vi "test.vi"() -> ()   [LabVIEW 2010]
uses:
  XImage/XImage.xctl
  classes/ImageCollection/ImageCollection/ImageCollection.lvclass
  XImage/ROI_mode_enum.ctl
  XImage/overlays_cluster.ctl
panel:
  in  "point radius":i32=5
  in  "Overlay":T1={"overlay array"=[{[[10, 10], [20, 30], [12, 45]]}], "overlay name"="test", "color (red)"=16711680, "overlay size"=3, "overlay type"=enum."crosshair"} {"overlay size" min=1}
  in  "size":cluster{"Width":u32, "Height":u32}
  in  "ROI mode":T2=enum."IMAQROIs"
  in  "overlay name":string
  in  "button:clear overlay":bool
  out "successful save?":bool
  in  "button:save ROIs":bool
  in  "button:load ROIs":bool
  in  "button:load image":bool
  out "has image loaded?":bool
  in  "enable numbering?":bool
  in  "ROI colour":u32(colorbox)=6618880
  in  "ROI Tools Palette visible":T3={"Zoom Tool"=TRUE, "Selection Tool"=TRUE, "Pan Tool"=TRUE, "Point Tool"=TRUE, "Line Tool"=TRUE, "Rectangle Tool"=TRUE, "Rotated Rectangle Tool"=TRUE, "Polyline Tool"=TRUE, "Polygon Tool"=TRUE, "Freehand Tool"=TRUE, "Closed Freehand Tool"=TRUE, "Ellipse Tool"=TRUE, "Annulus Tool"=TRUE}
  out "number of ROIs":i32
  in  "current frame index":i32
  out "number of images":i32
  in  "stop":bool
  in  "XImage":refnum<class "ImageCollection.lvclass">(xcontrol)
  # "Test panel for XImage"
  # "Overlay"
  # "ROIs"
  # "PointCollection"
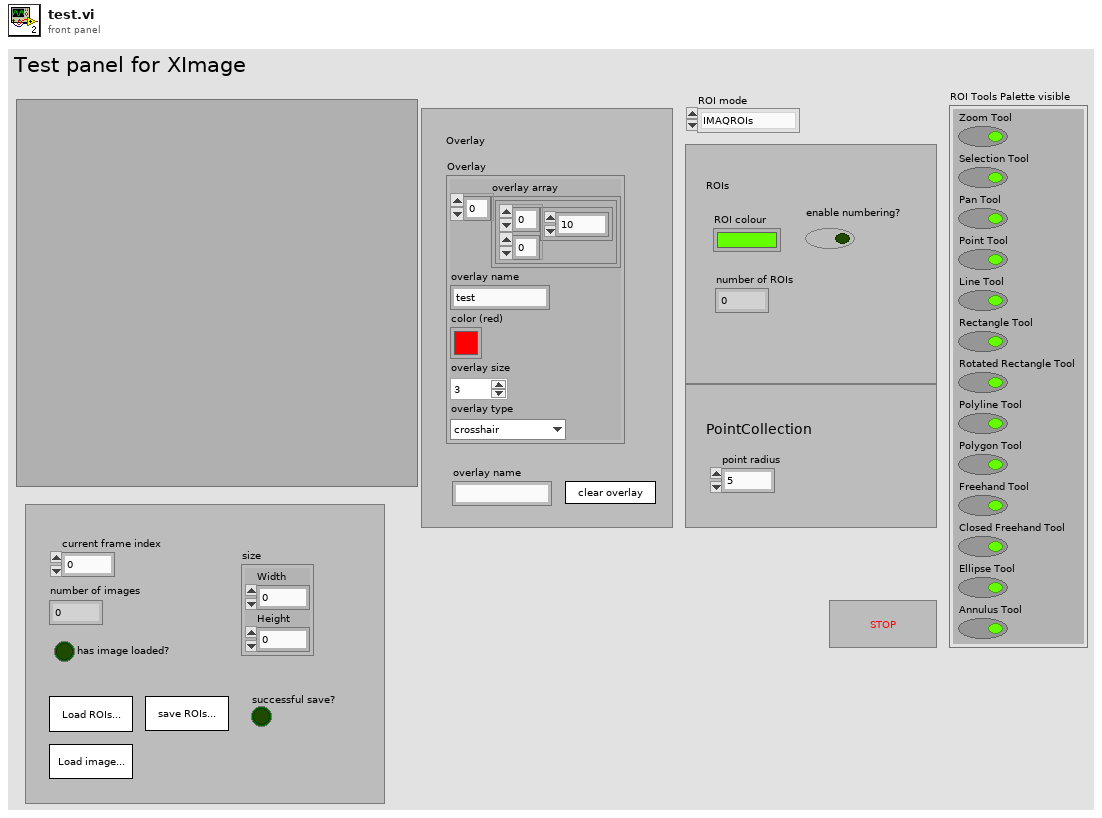
[diagram p1: front panel]
types:
  T1 = typedef "XImage.xctl/overlays_cluster.ctl" = cluster{"overlay array":cluster{i32[][]}[], "overlay name":string, "color (red)":u32, "overlay size":i32, "overlay type":enum16{"crosshair", "circle"}}
  T2 = typedef "XImage.xctl/ROI_mode_enum.ctl" = enum16{"none", "IMAQROIs", "PointCollection"}
  T3 = cluster{"Zoom Tool":bool, "Selection Tool":bool, "Pan Tool":bool, "Point Tool":bool, "Line Tool":bool, "Rectangle Tool":bool, "Rotated Rectangle Tool":bool, "Polyline Tool":bool, "Polygon Tool":bool, "Freehand Tool":bool, "Closed Freehand Tool":bool, "Ellipse Tool":bool, "Annulus Tool":bool}
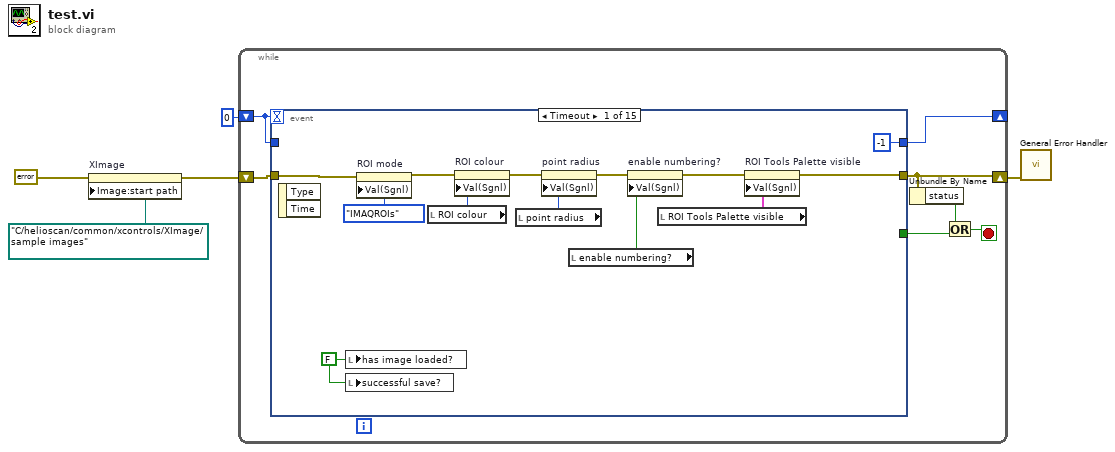
[diagram p0: block diagram]
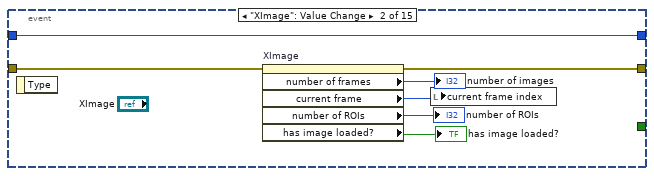
[diagram p2: hidden frame]
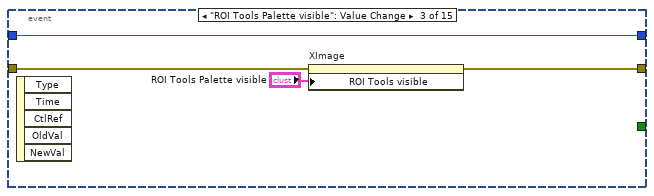
[diagram p3: hidden frame]
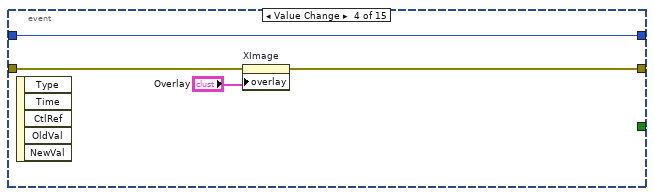
[diagram p4: hidden frame]
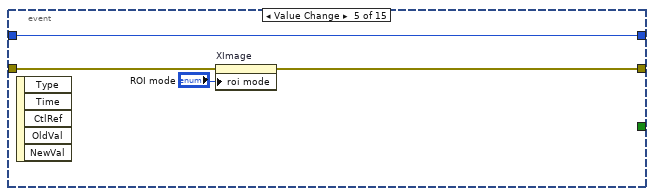
[diagram p5: hidden frame]
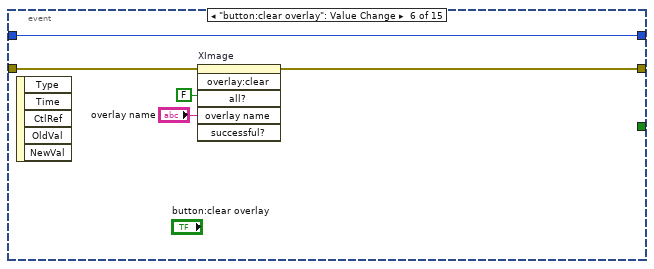
[diagram p6: hidden frame]
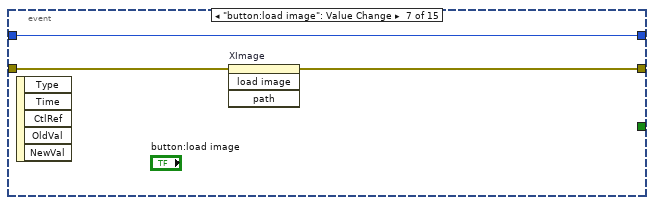
[diagram p7: hidden frame]
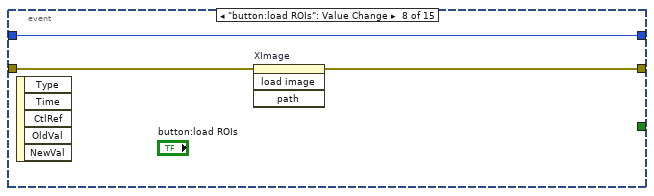
[diagram p8: hidden frame]
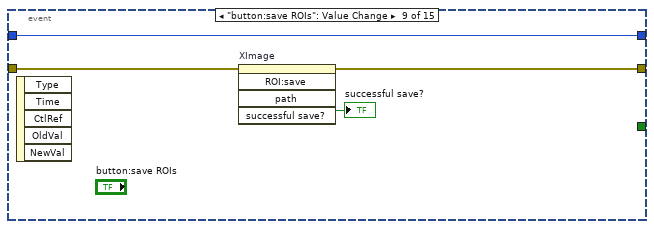
[diagram p9: hidden frame]
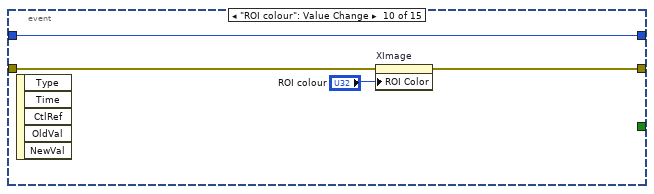
[diagram p10: hidden frame]
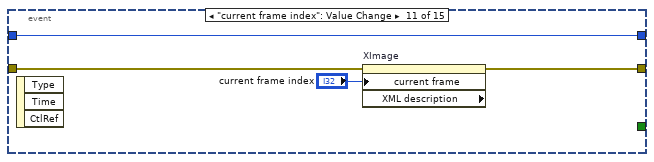
[diagram p11: hidden frame]
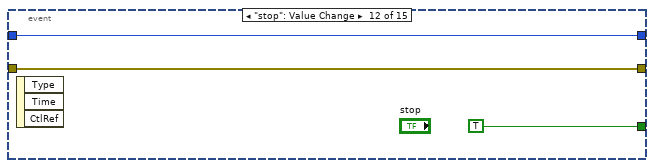
[diagram p12: hidden frame]
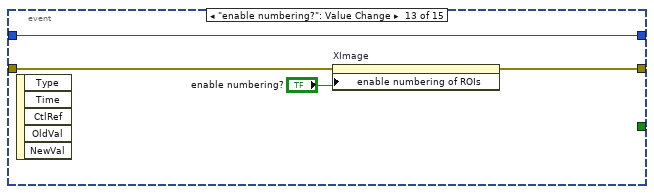
[diagram p13: hidden frame]
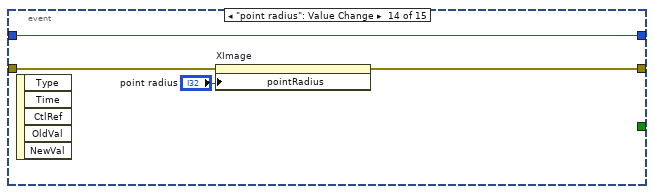
[diagram p14: hidden frame]
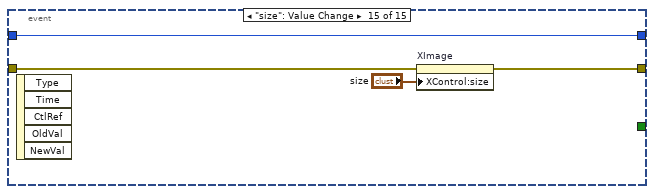
[diagram p15: hidden frame]
diagram:
  n1 = property on="XImage" class="XImage (strict)"(error in=errorcluster {"status"=FALSE, "code"=0, "source"=""} ("error out"), "Image:start path"=path "C:/helioscan/common/xcontrols/XImage/sample images") -> (error out=w3:errorcluster)  [unwired: 1 in, 1 out]
  n2 = while {
    shift-right: [w11] -> w5
    shift-left: w3 -> [w12]
    shift-right: [w6] -> _
    shift-left: 0 -> [w7]
    stop <- w9 stop-if-true
    n3 = event shown="[0] Timeout" {
      selector: _ -> [_ _ _ _ _ _ _ _ _ _ _ _ _ _ _]
      dyn-events: _ -> [_ _ _ _ _ _ _ _ _ _ _ _ _ _ _]
      timeout: w7 -> [_ _ _ _ _ _ _ _ _ _ _ _ _ _ _]
      tunnel: [w13 w31 w34 w39 w42 w45 w51 w54 w58 w62 w65 w70 w73 w75 w81] -> w11
      tunnel: w12 -> [w23 w32 w35 w37 w43 w49 w52 w55 w59 w63 w66 w70 w74 w76 w79]
      tunnel: [_ _ _ _ _ _ _ _ _ _ _ TRUE _ _ _] -> w8
      tunnel: w7 -> [_ w30 w36 w40 w41 w46 w50 w53 w56 w61 w64 w68 w72 w78 w82]
      tunnel: [-1 w30 w36 w40 w41 w46 w50 w53 w56 w61 w64 w68 w72 w78 w82] -> w6
      event Timeout {
        w22 = FALSE ("has image loaded?")
        n4 = event-data() -> ()  [unwired: 1 in, 2 out]
        n5 = local write "has image loaded?"(w22) -> ()
        n6 = local write "successful save?"(w22) -> ()
        n7 = property on="ROI mode" class="Enum (strict)"(error in=w23, "Val(Sgnl)"=ROI_mode_enum."IMAQROIs" ("Value (Signaling)")) -> (error out=w18:errorcluster)  [unwired: 1 in, 1 out]
        n8 = local read "ROI colour"() -> (w21:u32)
        n9 = property on="ROI colour" class="ColBox"(error in=w18, "Val(Sgnl)"=w21) -> (error out=w19:errorcluster)  [unwired: 1 in, 1 out]
        n10 = local read "point radius"() -> (w20:i32)
        n11 = property on="point radius" class="DigNum (strict)"(error in=w19, "Val(Sgnl)"=w20) -> (error out=w14:errorcluster)  [unwired: 1 in, 1 out]
        n12 = local read "enable numbering?"() -> (w16:bool)
        n13 = property on="enable numbering?" class="Bool (strict)"(error in=w14, "Val(Sgnl)"=w16) -> (error out=w15:errorcluster)  [unwired: 1 in, 1 out]
        n14 = local read "ROI Tools Palette visible"() -> (w17:T3)
        n15 = property on="ROI Tools Palette visible" class="Clust (strict)"(error in=w15, "Val(Sgnl)"=w17) -> (error out=w13:errorcluster)  [unwired: 1 in, 1 out]
      }
      event "XImage": Value Change {
        n16 = event-data() -> ()  [unwired: 1 in, 1 out]
        n17 = property on="XImage" class="XImage (strict)"(error in=w32) -> (error out=w31:errorcluster, "number of frames"=→"number of images":i32, "current frame"=w28:i32, "number of ROIs"=→"number of ROIs":i32, "has image loaded?"=→"has image loaded?":bool)  [unwired: 1 in, 1 out]
        n18 = local write "current frame index"(w28) -> ()
      }
      event "ROI Tools Palette visible": Value Change {
        n19 = event-data() -> ()  [unwired: 1 in, 5 out]
        n20 = property on="XImage" class="XImage (strict)"(error in=w35, "ROI Tools visible"="ROI Tools Palette visible") -> (error out=w34:errorcluster)  [unwired: 1 in, 1 out]
      }
      event Value Change {
        n21 = event-data() -> ()  [unwired: 1 in, 5 out]
        n22 = property on="XImage" class="XImage (strict)"(error in=w37, "overlay"="Overlay") -> (error out=w39:errorcluster)  [unwired: 1 in, 1 out]
      }
      event Value Change {
        n23 = event-data() -> ()  [unwired: 1 in, 5 out]
        n24 = property on="XImage" class="XImage (strict)"(error in=w43, "roi mode"="ROI mode") -> (error out=w42:errorcluster)  [unwired: 1 in, 1 out]
      }
      event "button:clear overlay": Value Change {
        n25 = event-data() -> ()  [unwired: 1 in, 5 out]
        n26 = invoke on="XImage" class="XImage (strict)" method="overlay:clear"(error in=w49, "all?"=FALSE, "overlay name"="overlay name") -> (error out=w45:errorcluster)  [unwired: 3 in, 5 out]
      }
      event "button:load image": Value Change {
        n27 = event-data() -> ()  [unwired: 1 in, 5 out]
        n28 = invoke on="XImage" class="XImage (strict)" method="load image"(error in=w52) -> (error out=w51:errorcluster)  [unwired: 3 in, 3 out]
      }
      event "button:load ROIs": Value Change {
        n29 = event-data() -> ()  [unwired: 1 in, 5 out]
        n30 = invoke on="XImage" class="XImage (strict)" method="load image"(error in=w55) -> (error out=w54:errorcluster)  [unwired: 3 in, 3 out]
      }
      event "button:save ROIs": Value Change {
        n31 = event-data() -> ()  [unwired: 1 in, 5 out]
        n32 = invoke on="XImage" class="XImage (strict)" method="ROI:save"(error in=w59) -> (error out=w58:errorcluster, "successful save?"=→"successful save?":bool)  [unwired: 4 in, 3 out]
      }
      event "ROI colour": Value Change {
        n33 = event-data() -> ()  [unwired: 1 in, 5 out]
        n34 = property on="XImage" class="XImage (strict)"(error in=w63, "ROI Color"="ROI colour") -> (error out=w62:errorcluster)  [unwired: 1 in, 1 out]
      }
      event "current frame index": Value Change {
        n35 = event-data() -> ()  [unwired: 1 in, 3 out]
        n36 = property on="XImage" class="XImage (strict)" props=["current frame", "XML description"](error in=w66, "current frame"="current frame index") -> (error out=w65:errorcluster)  [unwired: 1 in, 2 out]
      }
      event "stop": Value Change {
        n37 = event-data() -> ()  [unwired: 1 in, 3 out]
      }
      event "enable numbering?": Value Change {
        n38 = event-data() -> ()  [unwired: 1 in, 5 out]
        n39 = property on="XImage" class="XImage (strict)"(error in=w74, "enable numbering of ROIs"="enable numbering?") -> (error out=w73:errorcluster)  [unwired: 1 in, 1 out]
      }
      event "point radius": Value Change {
        n40 = event-data() -> ()  [unwired: 1 in, 5 out]
        n41 = property on="XImage" class="XImage (strict)"(error in=w76, "pointRadius"="point radius") -> (error out=w75:errorcluster)  [unwired: 1 in, 1 out]
      }
      event "size": Value Change {
        n42 = event-data() -> ()  [unwired: 1 in, 5 out]
        n43 = property on="XImage" class="XImage (strict)"(error in=w79, "XControl:size"="size") -> (error out=w81:errorcluster)  [unwired: 1 in, 1 out]
      }
    }
    n44 = Unbundle By Name(w11) -> ("status"=w10:bool)
    n45 = Or(x=w10, y=w8) -> (x .or. y?=w9:bool)
  }
  n46 = call <vilib>:"General Error Handler.vi"("error in (no error)"=w5) -> ()  [unwired: 10 in, 5 out]
